vi "Set Waveform Chart Plots Visibility.vi"(8 "error in (no error)":errorcluster, 9 "Plot.Visible":bool, 10 "Active Plot":u32[](array[numeric]), 11 "WaveformChart in":refnum<vi>) -> (0 "error out":errorcluster, 3 "WaveformChart out":refnum<vi>)   [LabVIEW 2020]
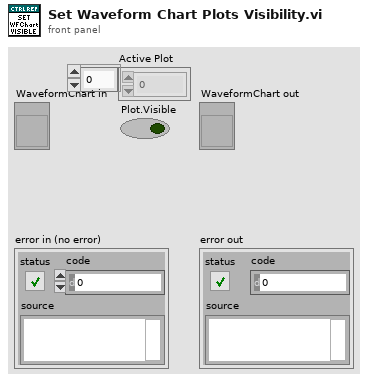
[diagram p1: front panel]
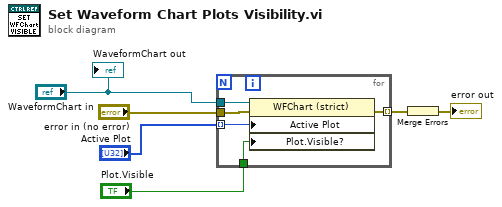
[diagram p0: block diagram]
diagram:
  n1 = for {
    tunnel: "WaveformChart in" -> [w11]
    tunnel: [w10] -> w5 mode=indexing
    tunnel: "error in (no error)" -> [w9]
    tunnel: "Active Plot" -> [w8] mode=indexing
    tunnel: "Plot.Visible" -> [w7]
    n2 = property on="Property Node" class="WFChart (strict)"(reference=w11, error in=w9, "Active Plot"=w8, "Plot.Visible?"=w7) -> (error out=w10:errorcluster)  [unwired: 1 out]
  }
  n3 = Merge Errors(w5) -> (→"error out":errorcluster)
  "WaveformChart out" <- "WaveformChart in"
